vi "czy proste sie przecinaja.vi"(1 "Równanie Prostej 2":dbl[](array[numeric]), 2 "Równanie Prostej 1":dbl[](array[numeric])) -> (0 "czy się przecinają ?":bool)   [LabVIEW 2016]
doc: "To subvi przyjumuje dwa równania prostych i zwraca punkt ich przecięcia lub bład(error output) jeśli takowy punkt nie istnieje"
uses:
  <vilib>/Analysis/NI_AALBase.lvlib
  <vilib>/Analysis/baseanly.llb/Real Determinant.vi
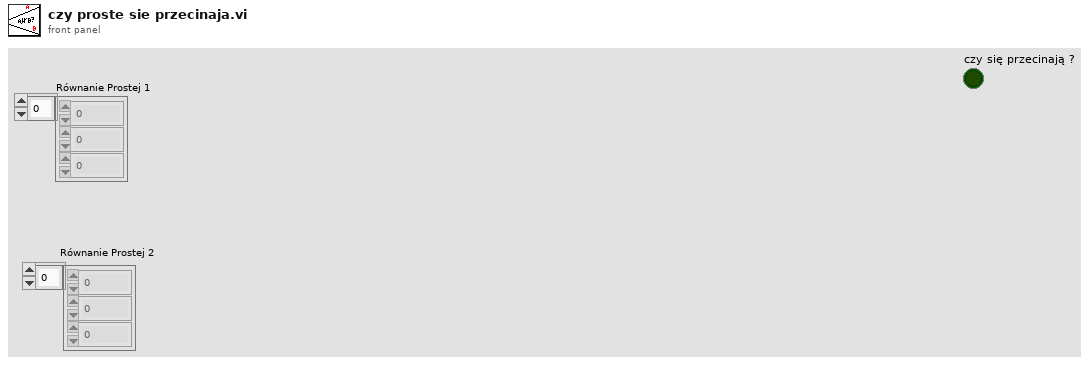
[diagram p1: front panel]
types:
  T1 = enum32{"General", "Positive Definite", "Lower Triangular", "Upper Triangular"}
  T2 = typedef "NI_Matrix.lvlib/RealMatrix.ctl" = dbl[][]
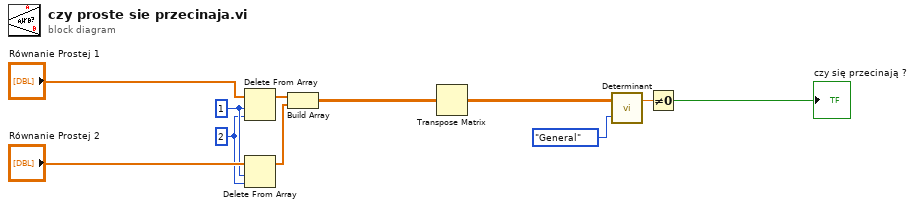
[diagram p0: block diagram]
diagram:
  w4 = 2 ("index")
  w5 = 1 ("length")
  n1 = Delete From Array(array="Równanie Prostej 1", length=w5, index=w4) -> (array with subset deleted=w9:dbl[])  [unwired: 1 out]
  n2 = Delete From Array(array="Równanie Prostej 2", length=w5, index=w4) -> (array with subset deleted=w8:dbl[])  [unwired: 1 out]
  n3 = Build Array(w9, w8) -> (w3:T2)
  n4 = Transpose Matrix(1:w3) -> (0:w2:T2)
  n5 = call-poly <vilib>:"Determinant.vi"("matrix type"=T1."General", "Input Matrix"=w2) -> ("determinant"=w7:dbl)  [unwired: 1 out]
  n6 = Not Equal To 0?(x=w7) -> (x != 0?=→"czy się przecinają ?":bool)
